vi "DUAL GAUGE-Get Set Point Status.vi"(8 "Fehler (Eingang)":errorcluster, 11 "Referenz in":refnum<visa-resource-name>) -> (0 "Cluster (Ausgang)":errorcluster, 1 "Set Point 3":u8(ring)=3 items=["off", "on"], 2 "Set Point 2":u8(ring)=3 items=["off", "on"], 3 "Referenz out":refnum<visa-resource-name>, 4 "Set Point 4":u8(ring)=3 items=["off", "on"], 5 "Set Point 1":u8(ring)=3 items=["off", "on"])   [LabVIEW 2010, in "Dual Gauge.lvlib"]
uses:
  Dual Gauge.lvlib
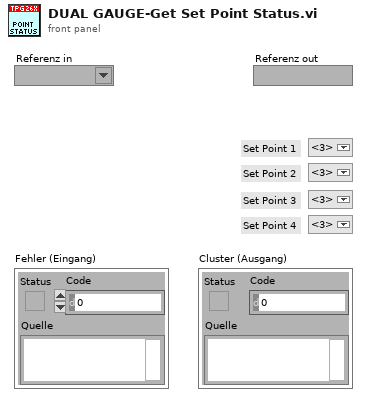
[diagram p1: front panel]
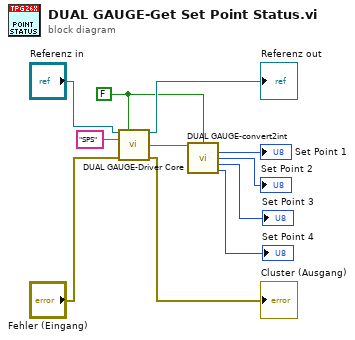
[diagram p0: block diagram]
diagram:
  w5 = FALSE ("Write/Read")
  n1 = call "DUAL GAUGE-Driver Core.vi"("Referenz in"="Referenz in", "Write/Read"=w5, "Command"="SPS", "Fehler (Eingang)"="Fehler (Eingang)") -> ("Referenz out"=→"Referenz out":refnum<visa-resource-name>, "String Out"=w6:string, "Cluster (Ausgang)"=→"Cluster (Ausgang)":errorcluster)  [unwired: 9 in]
  n2 = call "DUAL GAUGE-convert2int.vi"("String in"=w6, "W/R [W: Int in; Str out ]"=w5) -> ("Integer1 out"=→"Set Point 1":u8, "Integer2 out"=→"Set Point 2":u8, "Integer3 out"=→"Set Point 3":u8, "Integer4 out"=→"Set Point 4":u8)  [unwired: 9 in, 1 out]
